vi "Dashboard and Primary Interface.vi"() -> ()   [LabVIEW 2010]
uses:
  Z:/Samples/LabVIEW/Library/UnderAutomation.UniversalRobots.dll
  Library/UnderAutomation.UniversalRobots.dll
panel:
  out "Powered on":bool
  in  "Script to execute":string
  in  "Send script":bool
  out "Z":dbl
  out "Y":dbl
  out "X":dbl
  in  "Robot IP":string
  out "Connect error":errorcluster
  in  "Power off":bool
  in  "Power on\nRelease brake":bool
  out "Connected":bool
  out "License state":string
  in  "Connect":bool
  # "1. Connect to the robot"
  # "2. Dashboard"
  # "3. Primary Interface"
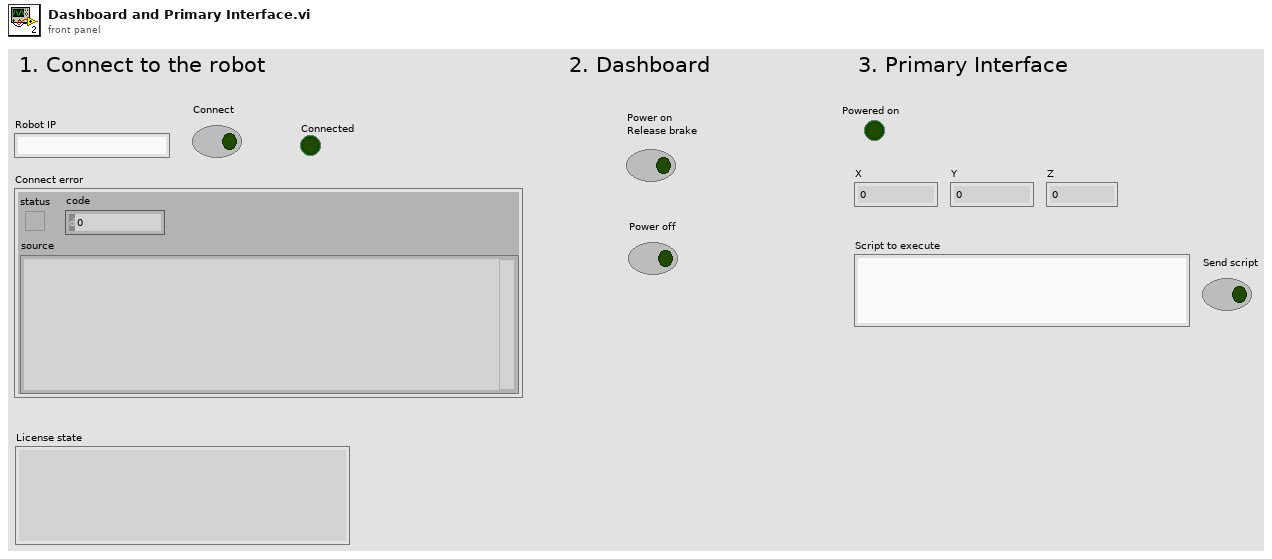
[diagram p1: front panel]
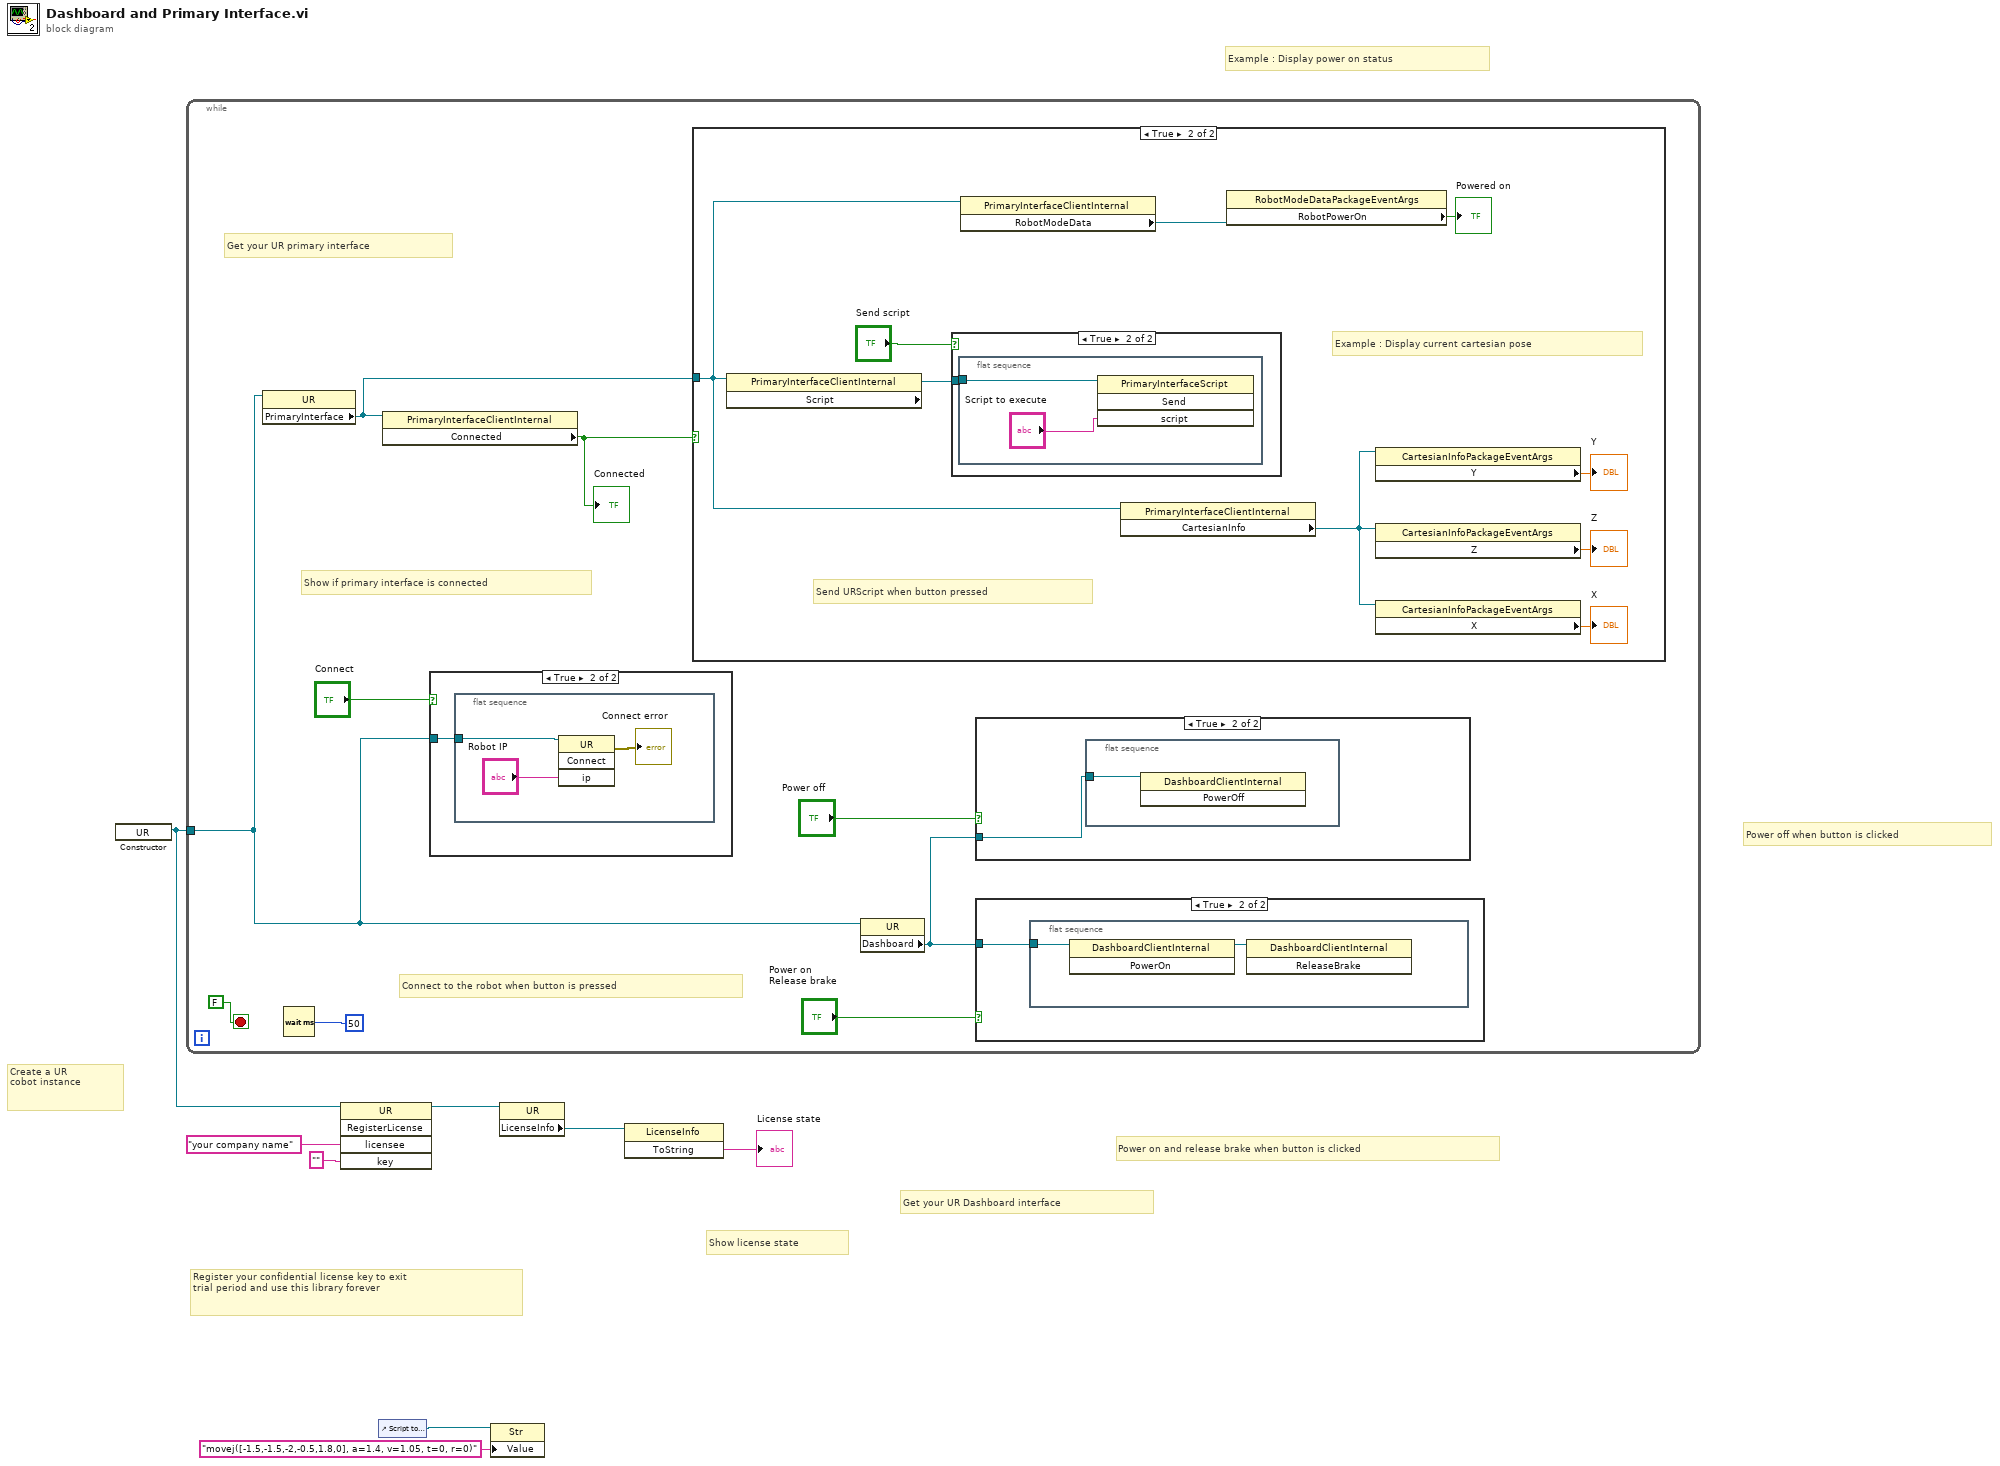
[diagram p0: block diagram]
diagram:
  # "Example : Display power on status"
  # "Create a UR\ncobot instance"
  # "Show license state"
  # "Register your confidential license key to exit\ntrial period and use this library forever"
  # "Power off when button is clicked"
  # "Power on and release brake when button is clicked"
  # "Get your UR Dashboard interface"
  n1 = constructor class="UR"() -> (reference out=w3:refnum<k24>)  [unwired: 3 in, 2 out]
  n2 = while {
    tunnel: w3 -> [w9]
    stop <- FALSE stop-if-true
    # "Connect to the robot when button is pressed"
    # "Show if primary interface is connected"
    # "Get your UR primary interface"
    n3 = property class="UR"(reference=w9) -> ("PrimaryInterface"=w12:refnum<k24>)  [unwired: 1 in, 2 out]
    n4 = Wait (ms)(milliseconds to wait=u32 50) -> ()  [unwired: 1 out]
    n5 = property class="PrimaryInterfaceClientInternal"(reference=w12) -> ("Connected"=w11:bool)  [unwired: 1 in, 2 out]
    "Connected" <- w11
    n6 = case shown="True" "Connect" {
      tunnel: w9 -> [_ w35]
      frame False {
      }
      frame True {
        n7 = flat-sequence {
          tunnel: w35 -> [w37]
          frame #0 {
            n8 = invoke class="UR" method="Connect"(reference=w37, "ip"="Robot IP") -> (error out=→"Connect error":errorcluster)  [unwired: 2 in, 3 out]
          }
        }
      }
    }
    n9 = case shown="True" w11 {
      tunnel: w12 -> [_ w18]
      frame False {
      }
      frame True {
        # "Send URScript when button pressed"
        # "Example : Display current cartesian pose"
        n10 = property class="PrimaryInterfaceClientInternal"(reference=w18) -> ("Script"=w25:refnum<k24>)  [unwired: 1 in, 2 out]
        n11 = case shown="True" "Send script" {
          tunnel: w25 -> [_ w27]
          frame False {
          }
          frame True {
            n12 = flat-sequence {
              tunnel: w27 -> [w29]
              frame #0 {
                n13 = invoke class="PrimaryInterfaceScript" method="Send"(reference=w29, "script"="Script to execute") -> ()  [unwired: 2 in, 4 out]
              }
            }
          }
        }
        n14 = property class="PrimaryInterfaceClientInternal"(reference=w18) -> ("RobotModeData"=w24:refnum<k24>)  [unwired: 1 in, 2 out]
        n15 = property class="PrimaryInterfaceClientInternal"(reference=w18) -> ("CartesianInfo"=w19:refnum<k24>)  [unwired: 1 in, 2 out]
        n16 = property class="RobotModeDataPackageEventArgs"(reference=w24) -> ("RobotPowerOn"=→"Powered on":bool)  [unwired: 1 in, 2 out]
        n17 = property class="CartesianInfoPackageEventArgs"(reference=w19) -> ("Y"=→"Y":dbl)  [unwired: 1 in, 2 out]
        n18 = property class="CartesianInfoPackageEventArgs"(reference=w19) -> ("Z"=→"Z":dbl)  [unwired: 1 in, 2 out]
        n19 = property class="CartesianInfoPackageEventArgs"(reference=w19) -> ("X"=→"X":dbl)  [unwired: 1 in, 2 out]
      }
    }
    n20 = property class="UR"(reference=w9) -> ("Dashboard"=w13:refnum<k24>)  [unwired: 1 in, 2 out]
    n21 = case shown="True" "Power off" {
      tunnel: w13 -> [_ w30]
      frame False {
      }
      frame True {
        n22 = flat-sequence {
          tunnel: w30 -> [w31]
          frame #0 {
            n23 = invoke class="DashboardClientInternal" method="PowerOff"(reference=w31) -> ()  [unwired: 2 in, 3 out]
          }
        }
      }
    }
    n24 = case shown="True" "Power on\nRelease brake" {
      tunnel: w13 -> [_ w32]
      frame False {
      }
      frame True {
        n25 = flat-sequence {
          tunnel: w32 -> [w34]
          frame #0 {
            n26 = invoke class="DashboardClientInternal" method="PowerOn"(reference=w34) -> (reference out=w33:refnum<k24>)  [unwired: 2 in, 2 out]
            n27 = invoke class="DashboardClientInternal" method="ReleaseBrake"(reference=w33) -> ()  [unwired: 2 in, 3 out]
          }
        }
      }
    }
  }
  n28 = invoke class="UR" method="RegisterLicense"(reference=w3, "licensee"="your company name", "key"="") -> (reference out=w5:refnum<k24>)  [unwired: 2 in, 4 out]
  n29 = control-ref of="Script to execute"() -> (w2:refnum<vi>)
  n30 = property class="Str"(reference=w2, "Value"="movej([-1.5,-1.5,-2,-0.5,1.8,0], a=1.4, v=1.05, t=0, r=0)") -> ()  [unwired: 1 in, 2 out]
  n31 = property class="UR"(reference=w5) -> ("LicenseInfo"=w4:refnum<k24>)  [unwired: 1 in, 2 out]
  n32 = invoke class="LicenseInfo" method="ToString"(reference=w4) -> ("ToString"=→"License state":string)  [unwired: 2 in, 2 out]
